vi "Send Message Reply.vi"(8 "error in (no error)":errorcluster, 9 "Reply Data":variant, 10 "Reply Channel":refnum<notifier>, 11 "Actor in":refnum<class "Actor.lvclass">) -> (0 "error out":errorcluster, 3 "Actor out":refnum<class "Actor.lvclass">)   [LabVIEW 2015, in "Actor.lvclass"]
uses:
  Actor.lvclass
  Messaging/Message/Message.lvclass
  Actor.lvclass/Actor.ctl
  Messaging/Message/Message.lvclass/Message.ctl
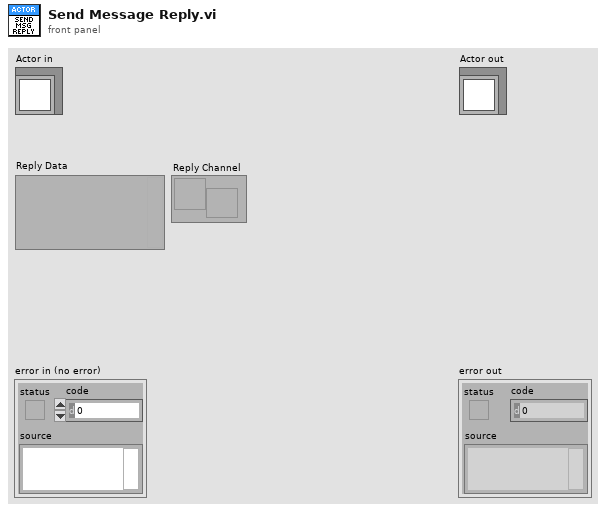
[diagram p1: front panel]
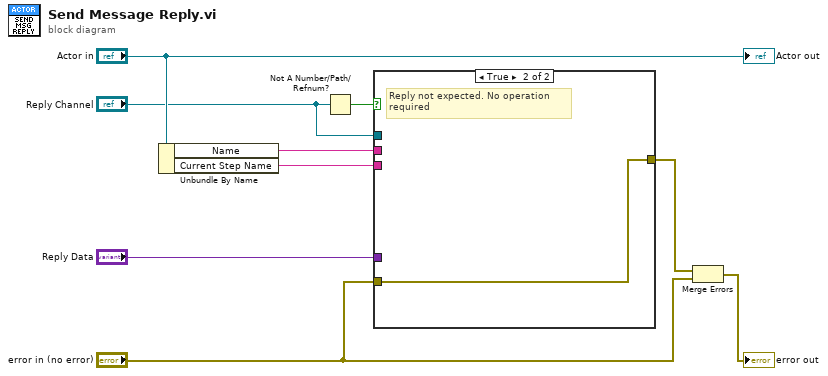
[diagram p0: block diagram]
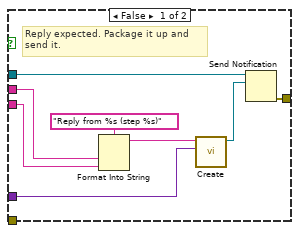
[diagram p2: hidden frame]
diagram:
  n1 = Unbundle By Name("Actor in") -> ("Name"=w3:string, "Current Step Name"=w2:string)
  n2 = Not A Number/Path/Refnum?(number/path/refnum="Reply Channel") -> (NaN/Path/Refnum?=w6:bool)
  n3 = case shown="True" w6 {
    tunnel: [w14 w18] -> w8
    tunnel: "Reply Channel" -> [w17 _]
    tunnel: "error in (no error)" -> [_ w18]
    tunnel: "Reply Data" -> [w16 _]
    tunnel: w3 -> [w11 _]
    tunnel: w2 -> [w10 _]
    frame False {
      # "Reply expected. Package it up and send it."
      n4 = Format Into String(format string="Reply from %s (step %s)", w11, w10) -> (resulting string=w12:string)  [unwired: 2 in, 1 out]
      n5 = call "Create.vi"("Data"=w16, "Name"=w12) -> ("Message out"=w15:refnum<class "Message.lvclass">)  [unwired: 8 in, 1 out]
      n6 = Send Notification(notification=w15, notifier=w17) -> (error out=w14:errorcluster)  [unwired: 1 in, 1 out]
    }
    frame True {
      # "Reply not expected. No operation required"
    }
  }
  n7 = Merge Errors(w8, "error in (no error)") -> (→"error out":errorcluster)
  "Actor out" <- "Actor in"
